vi "PH_Timing.Set GateGen.vi"(0 "i ref in":refnum<vi>, 5 "error in (no error)":errorcluster) -> (14 "i ref out":refnum<vi>, 19 "error out":errorcluster)   [LabVIEW 2014, in "PH_Timing.lvlib"]
doc: "This VI sets the GateGen configuration."
uses:
  PH_Timing.lvlib
  CSDigitalIO/BNC555/BNC555.lvlib
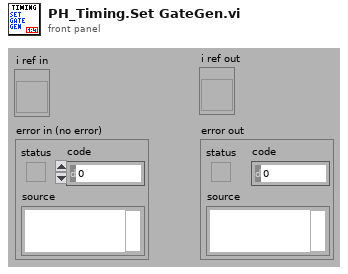
[diagram p1: front panel]
types:
  T1 = enum16{"Normal", "Single", "Burst", "Duty Cycle"}
  T2 = enum16{"Normal", "Single", "Burst", "Divide by N"}
  T3 = typedef "PH_Timing.lvlib/PH_Timing.i attribute.ctl" = cluster{"Sequencer":cluster{"linked?":bool, "Proc State":string, "Ref State":refnum<vi>}, "Gate Generator":cluster{"GD":cluster{"Device Status":T4, "linked?":bool}, "Settings":T5, "GUI Ref":refnum<vi>}, "Interlock Bypass":cluster{"Instancename":string, "Switch linked?":bool, "Device Status":T4, "Ref Status":refnum<vi>}, "Roughtuner":cluster{"Settings":T6, "GUI Ref":refnum<vi>, "GD":cluster{"Device Status":T4, "linked?":bool}}, "0,5Hz Gater":cluster{"Settings":T7, "GUI Ref":refnum<vi>, "GD":cluster{"Device Status":T4, "linked?":bool}}, "Slow Trigger":cluster{"Settings":T8, "GUI Ref":refnum<vi>, "Service ID Delay":i32, "Service ID Ext Trig":i32, "Wanted Settings":T8}, "Timing Mode":cluster{"Mode":T9, "GUI Ref":refnum<vi>, "Service ID T2":i32, "Service ID Mode":i32, "Wanted Mode":T9}, "ns Generator":cluster{"Settings":T10, "ns Generator Settings":refnum<vi>, "GD":cluster{"Device Status":T4, "linked?":bool}}, "Phase FEs":cluster{"Settings":T13, "GUI Ref":refnum<vi>, "Service ID Phase":i32, "Wanted Settings":T13}, "GD GUI Refs":refnum<vi>[], "Heads":T14[], "GUI Ref Delete":refnum<vi>}
  T4 = typedef "PH_StatusHandler.lvlib/PH_StatusHandler.Status.ctl" = i16
  T5 = typedef "PH_Timing.lvlib/PH_Timing.GateGen.ctl" = cluster{"Instance":string, "Channel Gate":i32, "Channel T2":i32, "Width Gate":dbl, "Width T2":dbl, "Delay Gate":dbl, "Delay T2":dbl, "Gate activ":bool, "T2 activ":bool, "System Mode":enum16{"Normal", "Single", "Burst", "Duty Cycle"}}
  T6 = typedef "PH_Timing.lvlib/PH_Timing.Roughtuner.ctl" = cluster{"Instance":string, "Phase PHELIX / UNILAC":cluster{"Channel":u16, "relative to":u16, "Delay [ms]":dbl}, "Pulse Length":cluster{"Channel":u16, "relative to":u16, "Delay [ms]":dbl}, "Trigger":cluster{"externally?":bool, "Rate [Hz]":dbl}}
  T7 = typedef "PH_Timing.lvlib/PH_Timing.0.5HzGater.ctl" = cluster{"Instance":string, "Channel ns FE Delay":i32, "Channel 0.5Hz":i32, "Width ns FE Delay":dbl, "Width 0.5Hz":dbl, "Delay ns FE Delay":dbl, "Delay 0.5Hz":dbl, "ns FE Delay active":bool, "0.5Hz activ":bool, "ns FE Delay inverted":bool, "0.5Hz inverted":bool}
  T8 = typedef "PH_Timing.lvlib/PH_Timing.Slow Trigger Settings.ctl" = cluster{"Delay":dbl, "externally triggered?":bool}
  T9 = typedef "PH_Timing.lvlib/PH_Timing.Timing Mode.ctl" = cluster{"T2":i16, "Modeselector":enum32{"10 Hz", "0.5 Hz", "Shot"}}
  T10 = typedef "PH_Timing.lvlib/PH_Timing.ns Generator.ctl" = cluster{"Instance":string, "Phase fs / ns FE":cluster{"Channel":T11, "Settings":T12}}
  T11 = typedef "Stanford Research DG645 - Driver.lvlib/Channel.ctl" = i32
  T12 = typedef "PH_SRDG645.lvlib/PH_SRDG645.Channel Settings.ctl" = cluster{"Delay [s]":dbl, "relative to":i32}
  T13 = typedef "PH_Timing.lvlib/PH_Timing.Phase FEs.ctl" = cluster{"Phase":dbl}
  T14 = typedef "PH_Timing.lvlib/PH_Timing.PU Data.ctl" = cluster{"linked?":bool, "Data":T15, "GD":cluster{"Device Status":T4, "linked?":bool}, "GUI Ref":refnum<vi>, "PU":T16}
  T15 = typedef "PH_Timing.lvlib/PH_Timing.PU Info.ctl" = cluster{"Act CH?":bool, "GD":string, "CH":i32, "Delay":dbl, "active":bool, "in Use?":bool}
  T16 = typedef "PH_PP_Common.lvlib/PH_PP_Common.PUs.ctl" = enum16{"no Info", "PA-19mm-1", "PA-19mm-2", "PA-45mm-PILC", "PA-45mm-MAIN", "MA-PU-1", "MA-PU-2", "MA-PU-3", "MA-PU-4", "MA-PU-5", "MA-PU-6", "MA-FR", "MA-PILC", "PA-45mm-DP"}
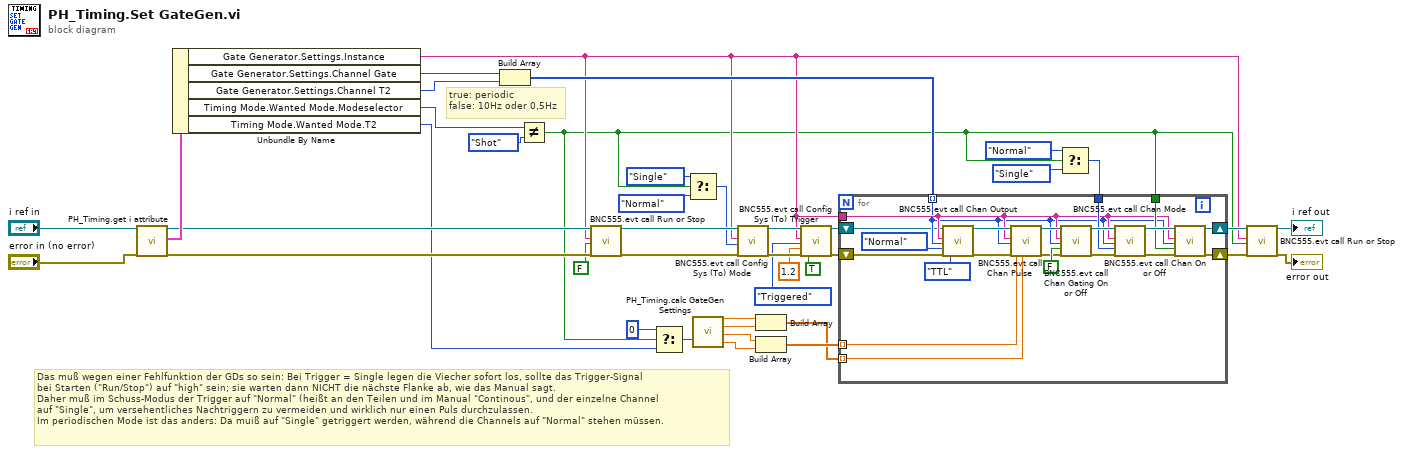
[diagram p0: block diagram]
diagram:
  # "true: periodic\nfalse: 10Hz oder 0,5Hz"
  # "Das muß wegen einer Fehlfunktion der GDs so sein: Bei Trigger = Single legen die Viecher sofort los, sollte das Trigger-Signal \nbei Starten (\"Run/Stop\") auf \"high\" sein; sie warten dann NICHT die nächste Flanke ab, wie das Manual sagt.\nDaher muß im Schuss-Modus der Trigger auf \"Normal\" (heißt an den Teilen und im Manual \"Continous\", und der einzelne Channel\nauf \"Single\", um versehentliches Nachtriggern zu vermeiden und wirklich nur einen Puls durchzulassen.\nIm periodischen Mode ist das anders: Da muiß auf \"Single\" getriggert werden, während die Channels auf \"Normal\" stehen müssen."
  n1 = call "PH_Timing.get i attribute.vi"("i ref in"="i ref in", "error in (no error)"="error in (no error)") -> ("i ref out"=w35:refnum<vi>, "i attribute"=w39:T3, "error out"=w36:errorcluster)  [unwired: 15 in]
  n2 = Unbundle By Name(w39) -> ("Gate Generator.Settings.Instance"=w5:string, "Gate Generator.Settings.Channel Gate"=w38:i32, "Gate Generator.Settings.Channel T2"=w37:i32, "Timing Mode.Wanted Mode.Modeselector"=w29:enum32{"10 Hz", "0.5 Hz", "Shot"}, "Timing Mode.Wanted Mode.T2"=w2:i16)
  n3 = Build Array(w38, w37) -> (w34:i32[])
  n4 = Not Equal?(x=w29, y=enum32{"10 Hz", "0.5 Hz", "Shot"}."Shot" ("Timing Mode.Mode.Modeselector")) -> (x != y?=w1:bool)
  n5 = call "BNC555.evt call Run or Stop.vi"("i ref in"=w35, "Generator Instance"=w5, "Start\\Stop"=FALSE ("Start\\Stop"), "error in (no error)"=w36) -> ("i ref out"=w12:refnum<vi>, "error out"=w11:errorcluster)  [unwired: 14 in]
  n6 = Select(t=i16 0, s=w1, f=w2) -> (s? t:f=w3:i16)
  n7 = Select(t=T1."Single" ("Mode"), s=w1, f=T1."Normal" ("Mode")) -> (s? t:f=w6:T1)
  n8 = call "PH_Timing.calc GateGen Settings.vi"("T2 [s]"=w3) -> ("Width Gate"=w27:dbl, "Width T2"=w26:dbl, "Delay Gate"=w25:dbl, "Delay T2"=w24:dbl)  [unwired: 23 in]
  n9 = call "BNC555.evt call Config Sys (To) Mode.vi"("i ref in"=w12, "Generator Instance"=w5, "Mode"=w6, "error in (no error)"=w11) -> ("i ref out"=w23:refnum<vi>, "error out"=w22:errorcluster)  [unwired: 14 in]
  n10 = Build Array(w27, w26) -> (w32:dbl[])
  n11 = Build Array(w25, w24) -> (w33:dbl[])
  n12 = call "BNC555.evt call Config Sys (To) Trigger.vi"("i ref in"=w23, "Generator Instance"=w5, "Mode"=enum16{"Disabled", "Triggered", "Gated"}."Triggered", "Trigger Level (2.5V)"=1.2 ("Trigger Level [V] (0.5)"), "error in (no error)"=w22, "Trigger Edge (T:Rising)"=TRUE) -> ("i ref out"=w21:refnum<vi>, "error out"=w20:errorcluster)  [unwired: 12 in]
  n13 = Select(t=T2."Normal" ("Mode (0:Normal)"), s=w1, f=T2."Single" ("Mode (0:Normal)")) -> (s? t:f=w16:T2)
  n14 = for {
    shift-right: [w55] -> w15
    shift-left: w21 -> [w43]
    shift-right: [w57] -> w14
    shift-left: w20 -> [w42]
    tunnel: w5 -> [w46]
    tunnel: w34 -> [w45] mode=indexing
    tunnel: w32 -> [w51] mode=indexing
    tunnel: w33 -> [w50] mode=indexing
    tunnel: w16 -> [w59]
    tunnel: w1 -> [w54]
    n15 = call "BNC555.evt call Chan Output.vi"("i ref in"=w43, "Generator Instance"=w46, "Channel"=w45, "Polarity (Normal)"=enum16{"Normal", "Complement", "Inverted"}."Normal", "error in (no error)"=w42, "Level (TTL)"=enum16{"TTL", "Adjustable", "35 Volt"}."TTL") -> ("i ref out"=w48:refnum<vi>, "error out"=w47:errorcluster)  [unwired: 12 in]
    n16 = call "BNC555.evt call Chan Pulse.vi"("i ref in"=w48, "Generator Instance"=w46, "Channel"=w45, "error in (no error)"=w47, "Delay"=w50, "Width"=w51) -> ("i ref out"=w53:refnum<vi>, "error out"=w52:errorcluster)  [unwired: 12 in]
    n17 = call "BNC555.evt call Chan Gating On or Off.vi"("i ref in"=w53, "Generator Instance"=w46, "Channel"=w45, "Gating State"=FALSE ("Gate enabled (false)"), "error in (no error)"=w52) -> ("i ref out"=w60:refnum<vi>, "error out"=w61:errorcluster)  [unwired: 13 in]
    n18 = call "BNC555.evt call Chan Mode.vi"("i ref in"=w60, "Generator Instance"=w46, "Channel"=w45, "Mode"=w59, "error in (no error)"=w61) -> ("i ref out"=w56:refnum<vi>, "error out"=w58:errorcluster)  [unwired: 13 in]
    n19 = call "BNC555.evt call Chan On or Off.vi"("i ref in"=w56, "Generator Instance"=w46, "Channel"=w45, "State"=w54, "error in (no error)"=w58) -> ("i ref out"=w55:refnum<vi>, "error out"=w57:errorcluster)  [unwired: 13 in]
  }
  n20 = call "BNC555.evt call Run or Stop.vi"("i ref in"=w15, "Generator Instance"=w5, "Start\\Stop"=w1, "error in (no error)"=w14) -> ("i ref out"=→"i ref out":refnum<vi>, "error out"=→"error out":errorcluster)  [unwired: 14 in]
